vi "pattern_generator.vi"(5 "fringe/stripe (fringe)":bool=TRUE, 6 "line position in px":i32, 7 "flip direction":bool, 8 "fringe number":dbl, 9 "phase":dbl(knob) min=0.0 max=6.28 scale=0.0..6.28) -> (1 "fringe pattern raw array":u8[][](array[numeric]), 2 "fringe pattern":T1(plugin-control))   [LabVIEW 2011]
doc: "Creates a fringe or a line pattern. \n\nfringe/stripe (default = fringe) - create fringe or line pattern\nphase - initial phase shift of the fringe pattern, starting at the left border\nfringe number - number of fringes that are created in the fringe pattern\nflip direction (default = false) - default are vertical fringes (=FALSE), if TRUE it will create horizontal fringes\nline position - postion of the created line, no meaning for created fringes"
uses:
  global_vars.vi
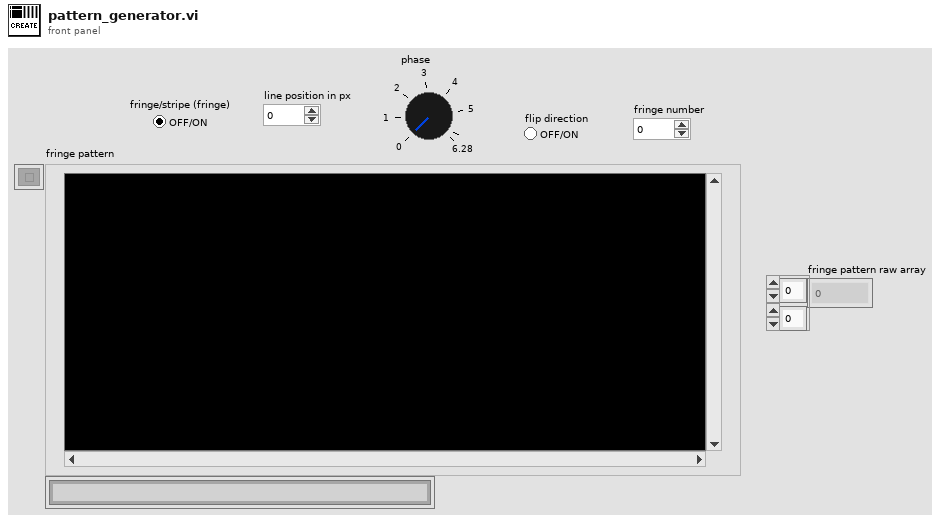
[diagram p1: front panel]
types:
  T1 = typedef "IMAQ Image.ctl" = refnum<image>
  T2 = typedef "Image Type" = u32
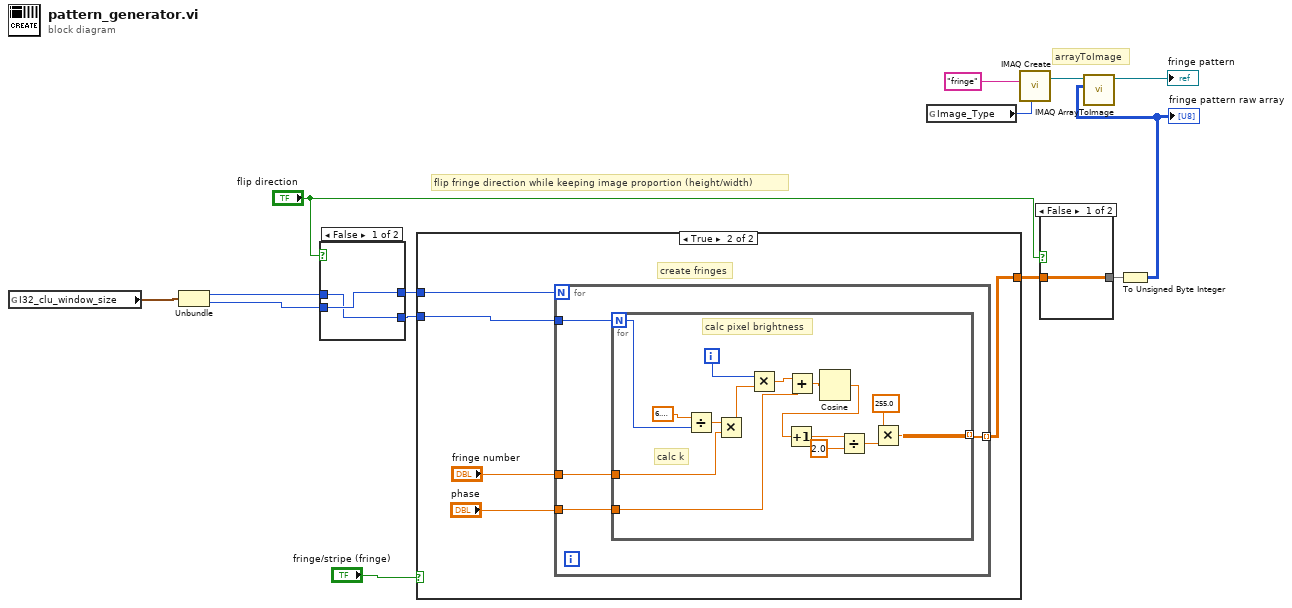
[diagram p0: block diagram]
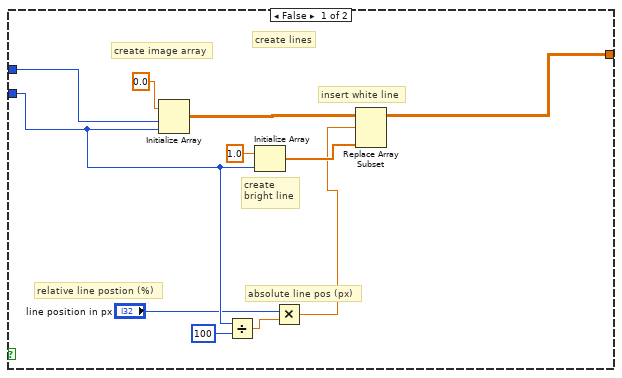
[diagram p2: hidden frame]
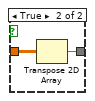
[diagram p4: hidden frame]
diagram:
  # "arrayToImage"
  # "flip fringe direction while keeping image proportion (height/width)"
  n1 = global read "global_vars.vi" "I32_clu_window_size"() -> (w4:cluster{"x Width(Px)":i32, "y height(Px)":i32})
  n2 = Unbundle(w4) -> ("x Width(Px)"=w6:i32, "y height(Px)"=w5:i32)
  n3 = case shown="False" "flip direction" {
    tunnel: w5 -> [w16 w18]
    tunnel: w6 -> [w15 w17]
    tunnel: [w15 w18] -> w11
    tunnel: [w16 w17] -> w10
    frame False {
    }
    frame True {
    }
  }
  n4 = case shown="True" "fringe/stripe (fringe)" {
    tunnel: [w24 w34] -> w12
    tunnel: w11 -> [w21 w33]
    tunnel: w10 -> [w27 w32]
    frame False {
      # "absolute line pos (px)"
      # "relative line postion (%)"
      # "create\nbright line"
      # "insert white line"
      # "create image array"
      # "create lines"
      n5 = Initialize Array(0.0 ("element"), w27, w21) -> (w28:dbl[][])
      n6 = Divide(x=w21, y=100) -> (x/y=w22:dbl)
      n7 = Initialize Array(1.0 ("element"), w21) -> (w25:dbl[])
      n8 = Multiply(x="line position in px", y=w22) -> (x*y=w20:dbl)
      n9 = Replace Array Subset(array=w28, new element=w25, index (row)=w20) -> (w24:dbl[][])  [unwired: 1 in]
    }
    frame True {
      # "create fringes"
      n10 = for {
        N: w32 -> [_]
        tunnel: [w38] -> w34 mode=indexing
        tunnel: w33 -> [w37]
        tunnel: "phase" -> [w36]
        tunnel: "fringe number" -> [w35]
        n11 = for {
          N: w37 -> [w45]
          tunnel: [w39] -> w38 mode=indexing
          tunnel: w35 -> [w49]
          tunnel: w36 -> [w47]
          i -> [w52]
          # "calc pixel brightness"
          # "calc k"
          n12 = Divide(x=6.283185307179586, y=w45) -> (x/y=w51:dbl)
          n13 = Multiply(x=w51, y=w49) -> (x*y=w50:dbl)
          n14 = Multiply(x=w52, y=w50) -> (x*y=w48:dbl)
          n15 = Add(x=w48, y=w47) -> (x+y=w46:dbl)
          n16 = Cosine(x=w46) -> (cos(x)=w44:dbl)
          n17 = Increment(x=w44) -> (x+1=w43:dbl)
          n18 = Divide(x=w43, y=2.0) -> (x/y=w41:dbl)
          n19 = Multiply(x=255.0, y=w41) -> (x*y=w39:dbl)
        }
      }
    }
  }
  n20 = global read "global_vars.vi" "Image_Type"() -> (w3:T2)
  n21 = call "IMAQ Create"("Image Name"="fringe", "Image Type"=w3) -> ("New Image"=w8:T1)  [unwired: 2 in, 2 out]
  n22 = case shown="False" "flip direction" {
    tunnel: w12 -> [w54 w56]
    tunnel: [w54 w55] -> w2
    frame False {
    }
    frame True {
      n23 = Transpose 2D Array(2D array=w56) -> (transposed array=w55:dbl[][])
    }
  }
  n24 = To Unsigned Byte Integer(number=w2) -> (unsigned 8bit integer=w1:u8[][])
  "fringe pattern raw array" <- w1
  n25 = call "IMAQ ArrayToImage"("Image Pixels (U8)"=w1, "Image"=w8) -> ("Image Out"=→"fringe pattern":T1)  [unwired: 8 in, 1 out]
